vi "Case_Structure.vi"() -> ()   [LabVIEW 2020]
panel:
  in  "stop":bool
  out "Resultado":dbl
  in  "Numero 2":dbl
  in  "Numero 1":dbl
  in  "Boolean":bool
  # "SUMA"
  # "RESTA"
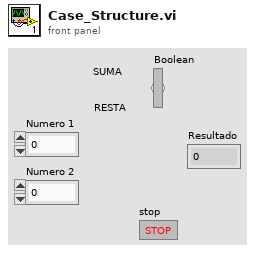
[diagram p1: front panel]
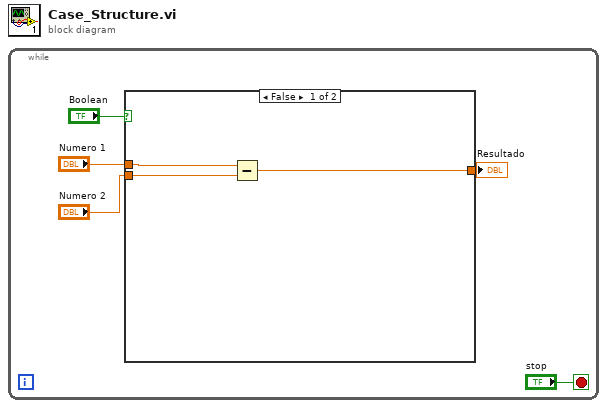
[diagram p0: block diagram]
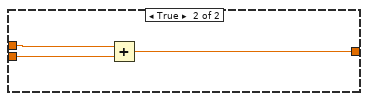
[diagram p2: hidden frame]
diagram:
  n1 = while {
    stop <- "stop" stop-if-true
    n2 = case shown="False" "Boolean" {
      tunnel: "Numero 1" -> [w7 w11]
      tunnel: "Numero 2" -> [w8 w10]
      tunnel: [w6 w9] -> w2
      frame False {
        n3 = Subtract(x=w7, y=w8) -> (x-y=w6:dbl)
      }
      frame True {
        n4 = Add(x=w11, y=w10) -> (x+y=w9:dbl)
      }
    }
    "Resultado" <- w2
  }
